vi "DecisitionMaker.vi"(0 "CameraControllerParameters.Diagnostics":T1, 2 "Histogram Report":T2, 5 "error in (no error)":errorcluster) -> (11 "Dust present":bool, 13 "Black Spots":bool, 14 "Diagnostics Passed":bool, 15 "Waveform Graph":u32[](graph), 16 "Dust Percentage":dbl, 18 "Range Percentage":dbl[](array[numeric]), 19 "error out":errorcluster)   [LabVIEW 2019]
uses:
  Camera Controller/Camera Controller Actor/TypeDef/CameraControllerParameters.ctl
  Camera Controller/Camera Controller Actor/Camera Controller.lvclass
panel:
  out "Black spot":u32
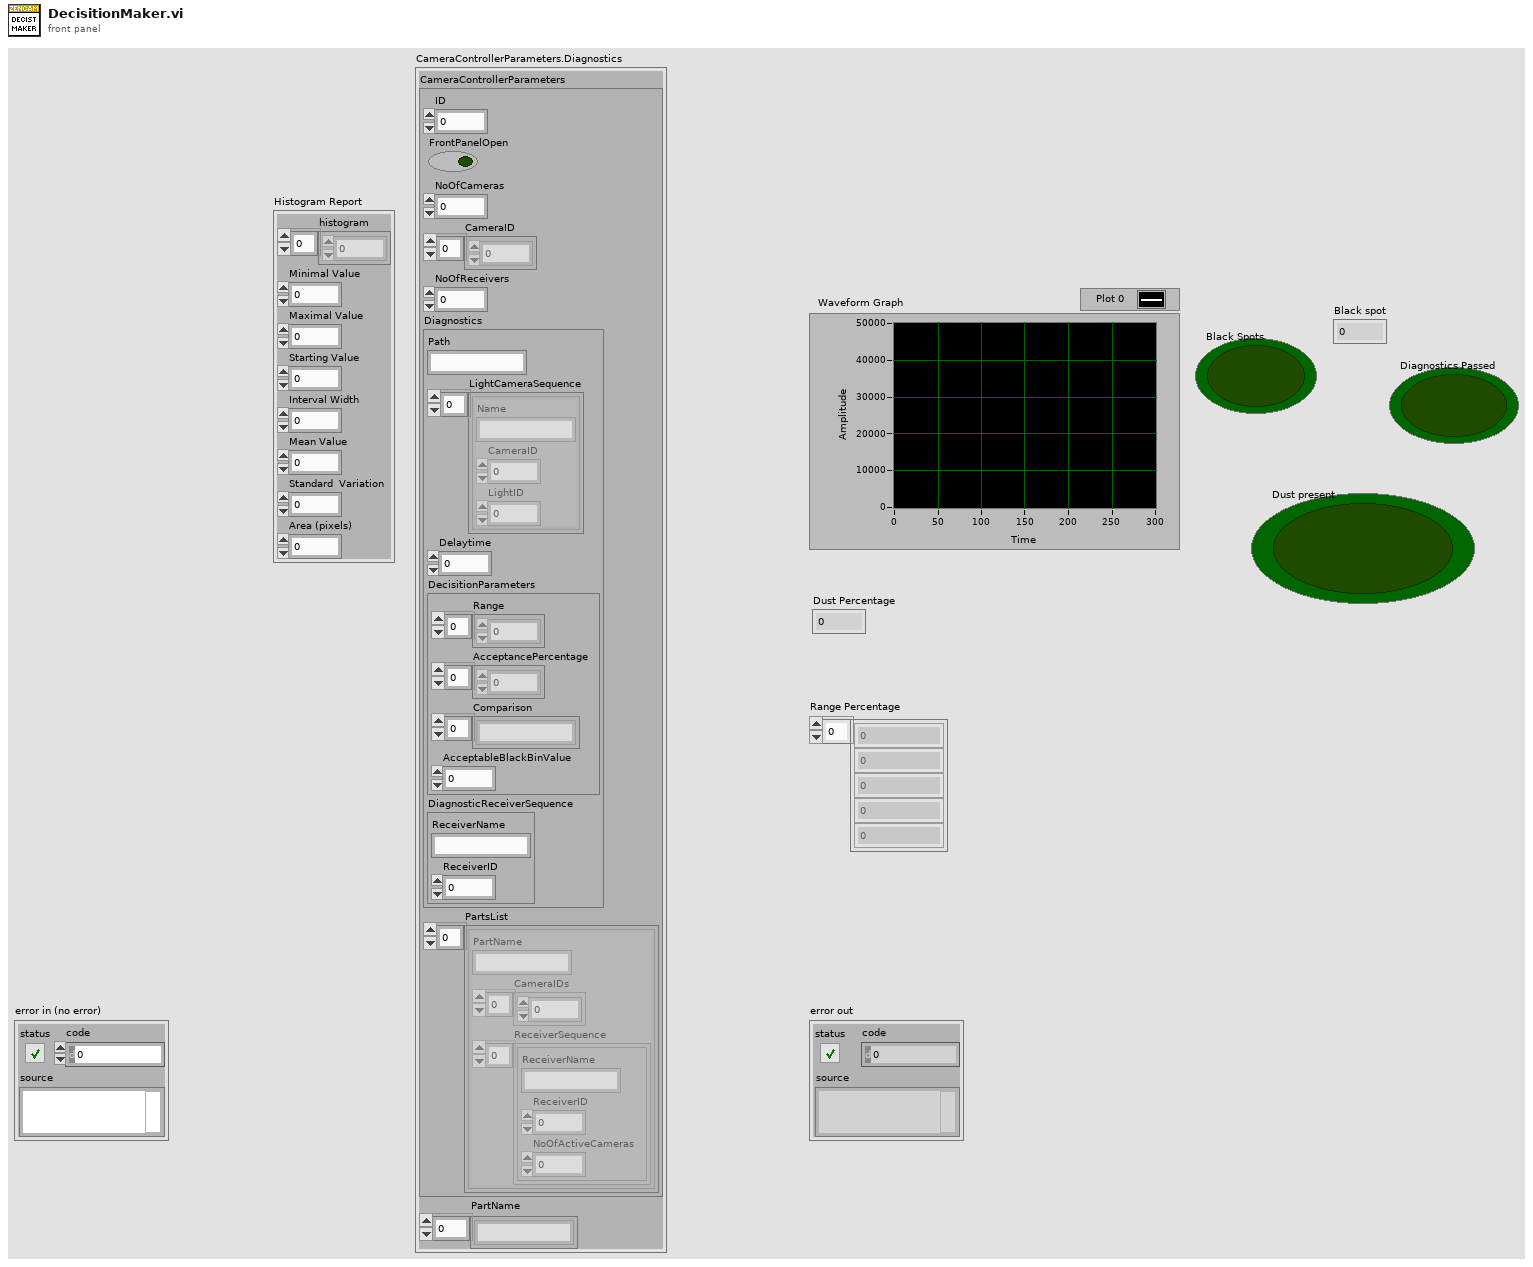
[diagram p1: front panel]
types:
  T1 = typedef "Camera Controller.lvlib/Camera Controller.lvclass/CameraControllerParameters.ctl" = cluster{"CameraControllerParameters":cluster{"ID":i32, "FrontPanelOpen":bool, "NoOfCameras":i32, "CameraID":i32[], "NoOfReceivers":i32, "Diagnostics":cluster{"Path":string, "LightCameraSequence":cluster{"Name":string, "CameraID":i32, "LightID":i32}[], "Delaytime":dbl, "DecisitionParameters":cluster{"Range":i32[], "AcceptancePercentage":i32[], "Comparison":string[], "AcceptableBlackBinValue":i32}, "DiagnosticReceiverSequence":cluster{"ReceiverName":string, "ReceiverID":i32}}, "PartsList":cluster{"PartName":string, "CameraIDs":i32[], "ReceiverSequence":cluster{"ReceiverName":string, "ReceiverID":i32, "NoOfActiveCameras":i32}[]}[]}, "PartName":string[]}
  T2 = cluster{"histogram":u32[], "Minimal Value":sgl, "Maximal Value":sgl, "Starting Value":sgl, "Interval Width":sgl, "Mean Value":sgl, "Standard  Variation":sgl, "Area (pixels)":i32}
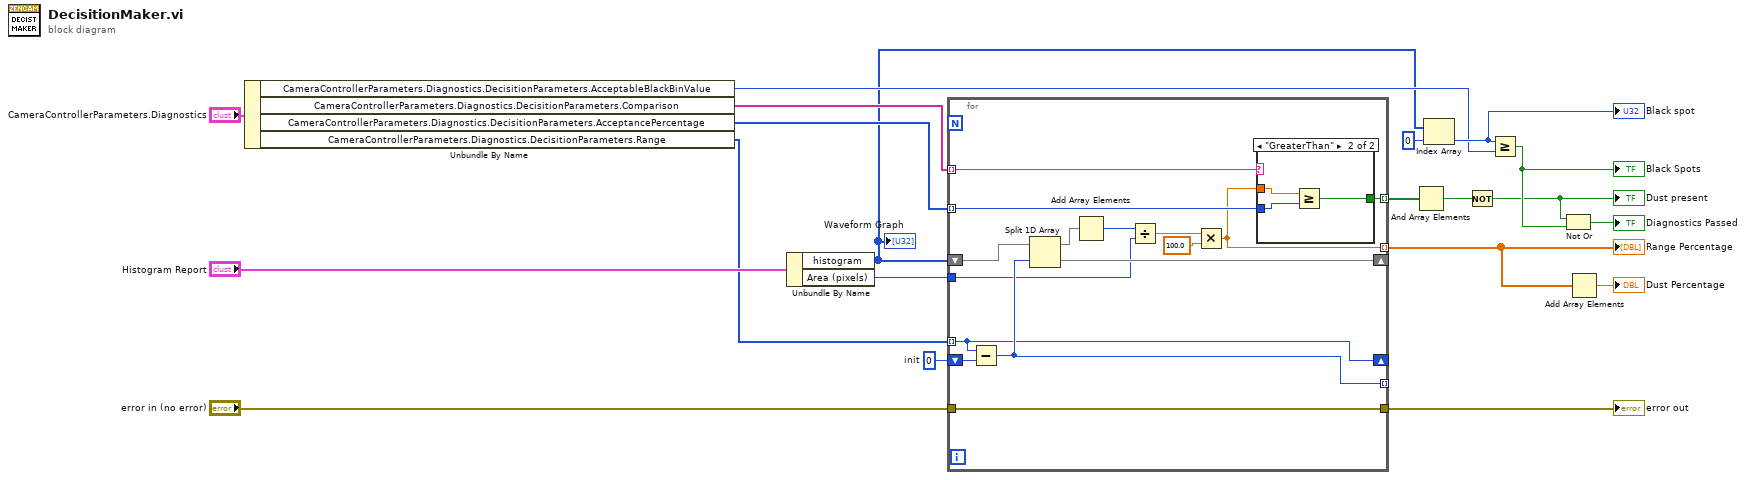
[diagram p0: block diagram]
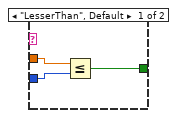
[diagram p2: hidden frame]
diagram:
  w20 = 0  # init
  n1 = Unbundle By Name("CameraControllerParameters.Diagnostics") -> ("CameraControllerParameters.Diagnostics.DecisitionParameters.AcceptableBlackBinValue"=w2:i32, "CameraControllerParameters.Diagnostics.DecisitionParameters.Comparison"=w15:string[], "CameraControllerParameters.Diagnostics.DecisitionParameters.AcceptancePercentage"=w14:i32[], "CameraControllerParameters.Diagnostics.DecisitionParameters.Range"=w13:i32[])
  n2 = Unbundle By Name("Histogram Report") -> ("histogram"=w1:u32[], "Area (pixels)"=w19:i32)
  "Waveform Graph" <- w1
  n3 = for {
    tunnel: w13 -> [w30] mode=indexing
    shift-right: [w30] -> _
    shift-left: w20 -> [w34]
    shift-right: [w32] -> _
    shift-left: w1 -> [w35]
    tunnel: [w31] -> _ mode=indexing
    tunnel: w19 -> [w29]
    tunnel: [w25] -> w10 mode=indexing
    tunnel: w14 -> [w26] mode=indexing
    tunnel: [w24] -> w18 mode=indexing
    tunnel: w15 -> [w23] mode=indexing
    tunnel: "error in (no error)" -> [w22]
    tunnel: [w22] -> w11
    n4 = Subtract(x=w30, y=w34) -> (x-y=w31:i32)
    n5 = Split 1D Array(array=w35, index=w31) -> (first subarray=w33:u32[], second subarray=w32:u32[])
    n6 = Add Array Elements(numeric array=w33) -> (sum=w21:u32)
    n7 = Divide(x=w21, y=w29) -> (x/y=w28:dbl)
    n8 = Multiply(x=w28, y=100.0 ("Percentage factor")) -> (x*y=w25:dbl)
    n9 = case shown="\"GreaterThan\"" w23 {
      tunnel: w26 -> [w36 w41]
      tunnel: w25 -> [w37 w40]
      tunnel: [w38 w39] -> w24
      frame "LesserThan", Default {
        n10 = Less Or Equal?(x=w37, y=w36) -> (x <= y?=w38:bool)
      }
      frame "GreaterThan" {
        n11 = Greater Or Equal?(x=w40, y=w41) -> (x >= y?=w39:bool)
      }
    }
  }
  "Range Percentage" <- w10
  "error out" <- w11
  n12 = And Array Elements(Boolean array=w18) -> (logical AND=w17:bool)
  n13 = Index Array(array=w1, index=0) -> (element=w6:u32)
  "Black spot" <- w6
  n14 = Not(x=w17) -> (.not. x?=w3:bool)
  "Dust present" <- w3
  n15 = Greater Or Equal?(x=w6, y=w2) -> (x >= y?=w4:bool)
  "Black Spots" <- w4
  n16 = Not Or(1:w4, 2:w3) -> (0:→"Diagnostics Passed":bool)
  n17 = Add Array Elements(numeric array=w10) -> (sum=→"Dust Percentage":dbl)
